vi "RemoteControl.ZMQ.TestServer.vi"   [LabVIEW 2019, in "RemoteControl.ZMQ.lvlib" / "RemoteControl.ZMQ.lvclass"]
uses:
  RemoteControl.ZMQ.lvclass
  C:/Program Files/National Instruments/LabVIEW 2019/user.lib/LevyLab/RemoteControl/RemoteControl/RemoteControl.lvclass
  <userlib>/LevyLab/RemoteControl/RemoteControl/RemoteControl.lvclass
panel:
  # "Run Me"
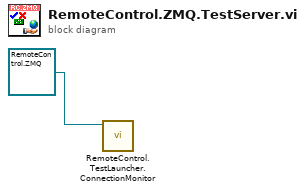
[diagram p0: block diagram]
diagram:
  n1 = call <userlib>:"RemoteControl.TestLauncher.ConnectionMonitor.vi"("RemoteControl in"=refnum<class "RemoteControl.ZMQ.lvclass"> refnum ("RemoteControl.ZMQ.lvlib:RemoteControl.ZMQ.lvclass")) -> ()  [unwired: 10 in, 1 out]
